vi "ATS_AsyncDMA_cFlags.vi"(7 "DeviceIn":i32, 8 "ReadSamples":T1, 10 "cFlags_Options":T2, 11 "Start Now / Wait":bool) -> (3 "cFlags_Out":u32 format="%.0x", 5 "DeviceOut":i32)   [LabVIEW 2010]
doc: "_____AlazarTech, Scope_____\n\nCreate the cFlags parameter on the StartAutoDMA and Asynchronous DMA transfer mode."
uses:
  ATS_ctl/ATS_AsyncDMA_cFlags_Opt.ctl
  ATS_ctl/ATS_ReadSamples.ctl
  ATS_ctl/ATS_Spec_Selector.ctl
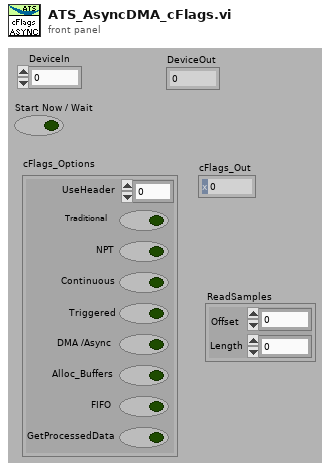
[diagram p1: front panel]
types:
  T1 = typedef "ATS_ReadSamples.ctl" = cluster{"Offset":i32, "Length":u32}
  T2 = typedef "ATS_AsyncDMA_cFlags_Opt.ctl" = cluster{"UseHeader":u32, "Traditional":bool, "NPT":bool, "Continuous":bool, "Triggered":bool, "DMA /Async":bool, "Alloc_Buffers":bool, "FIFO":bool, "GetProcessedData":bool}
  T3 = typedef "ATS_Spec_Selector.ctl" = enum16{"None", "ClckSource", "ClckEdge", "ClckRate", "InputRange", "InputCoupling", "Impedance", "Bandwidth", "AsyncDMA", "Memory", "ExtTrigCoupling", "ExtTrigRange", "AUX_IO_Trig", "AUX_IO_Slope", "Trigger_Source"}
  T4 = typedef "ATS_Global_Specs_Ctrl.ctl" = cluster{"ClckSource":cluster{"Internal":bool, "External":bool, "Medium Ext.":bool, "Slow Ext.":bool, "Ext. AC":bool, "Ext. DC":bool, "Ext. (PLL)":bool}, "ClckRate":cluster{"1 kS/s":bool, "2 kS/s":bool, "5 kS/s":bool, "10 kS/s":bool, "20 kS/s":bool, "50 kS/s":bool, "100 kS/s":bool, "200 kS/s":bool, "500 kS/s":bool, "1 MS/s":bool, "2 MS/s":bool, "5 MS/s":bool, "10 MS/s":bool, "20 MS/s":bool, "25 MS/s":bool, "50 MS/s":bool, "100 MS/s":bool, "125 MS/s":bool, "160 MS/s":bool, "180 MS/s":bool, "200 MS/s":bool, "250 MS/s":bool, "500 MS/s":bool, "1 GS/s":bool}, "ClckEdge":cluster{"Rising":bool, "Falling":bool}, "InputCoupling":cluster{"AC":bool, "DC":bool}, "InputRange":cluster{"20mV":bool, "40mV":bool, "50mV":bool, "80mV":bool, "100mV":bool, "200mV":bool, "400mV":bool, "500mV":bool, "800mV":bool, "1 V":bool, "2 V":bool, "4 V":bool, "5 V":bool, "8 V":bool, "10 V":bool, "16 V":bool, "20 V":bool, "40 V":bool, "HiFi":bool, "1.25 V":bool}, "Impedance":cluster{"1M ohms":bool, "50 ohms":bool, "300 ohms":bool}, "Bandwidth":cluster{"Full":bool, "Reduce":bool}, "RangeLim(50)":string, "AsyncDMA":cluster{"OnBoard":bool, "FPGA":bool}, "Memory":cluster{"VerifMem":bool, "HighMem":bool, "Combine":bool, "HighRecord":bool}, "ExtTrigCoupling":cluster{"AC":bool, "DC":bool}, "ExtTrigRange":cluster{"1 V":bool, "5 V":bool, "\nTTL":bool}, "AUX_IO_Trig":cluster{"Trig_Out":bool, "Trig_In":bool}, "AUX_IO_Slope":cluster{"Rising":bool, "Falling":bool}, "MaxPretrig":cluster{"MEM":u32, "FIFO":u32}, "AUX_I/O_Trig":cluster{"OUT_Trigger":bool, "OUT_PACER":bool, "OUT_BUSY":bool, "OUT_CLOCK":bool, "OUT_RESERVED":bool, "OUT_CAPTURE_ALMOST_DONE":bool, "OUT_AUXILIARY":bool, "OUT_SERIAL_DATA":bool, "IN_TRIGGER_ENABLE":bool, "IN_DIGITAL_TRIGGER":bool, "IN_GATE":bool, "IN_CAPTURE_ON_DEMAND":bool, "IN_RESET_TIMESTAMP":bool, "IN_SLOW_EXTERNAL_CLOCK":bool, "INPUT_AUXILIARY":bool, "INPUT_SERIAL_DATA":bool}, "ChannelsPerBoard":u8}
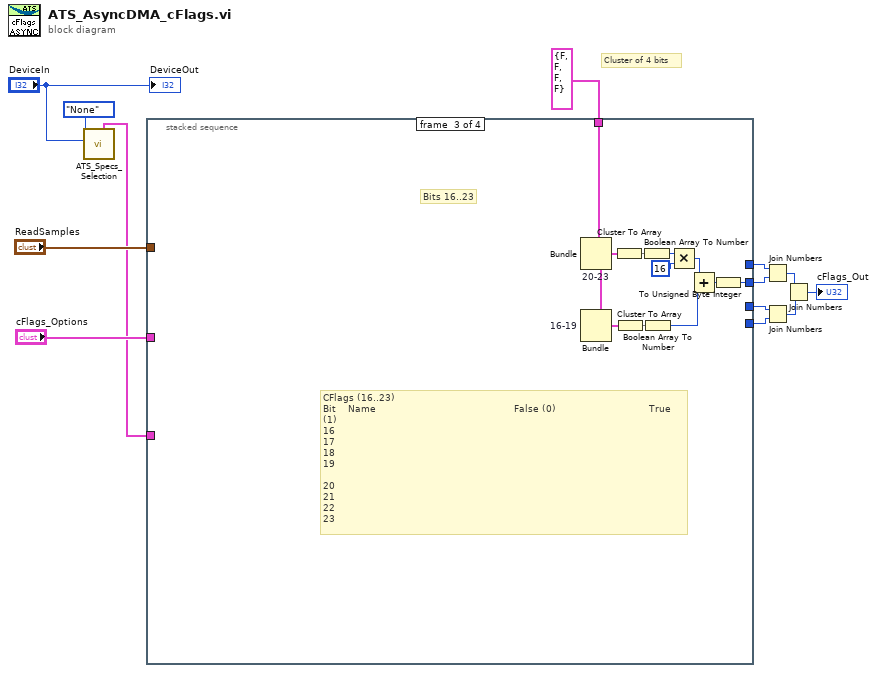
[diagram p0: block diagram]
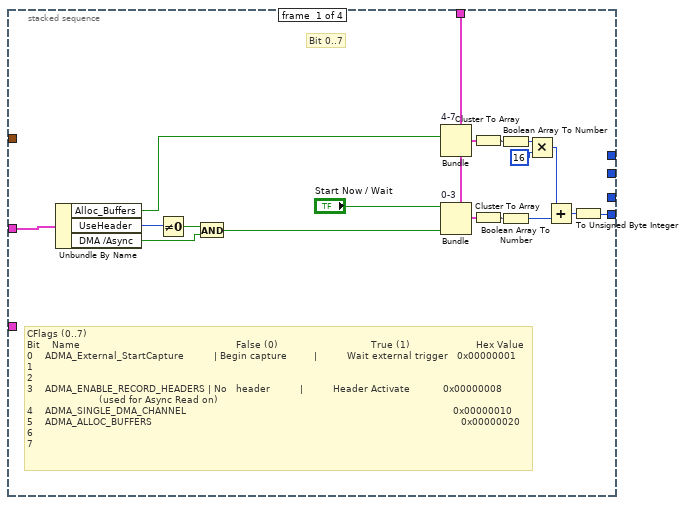
[diagram p2: hidden frame]
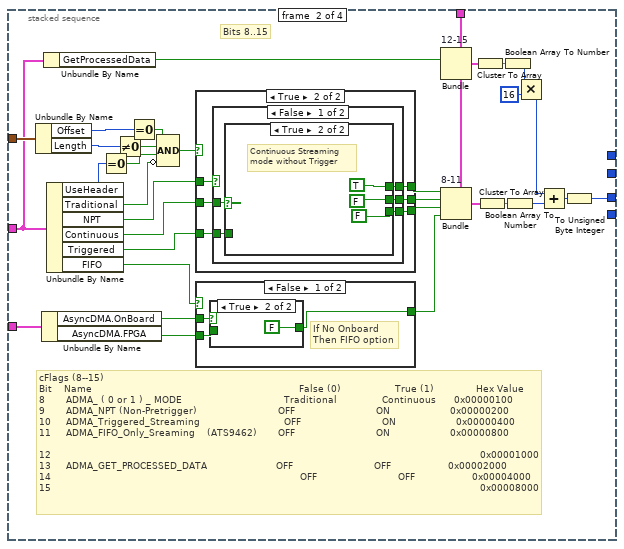
[diagram p3: hidden frame]
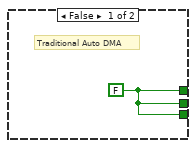
[diagram p6: hidden frame]
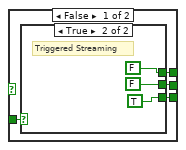
[diagram p7: hidden frame]
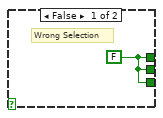
[diagram p8: hidden frame]
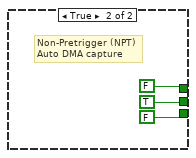
[diagram p9: hidden frame]
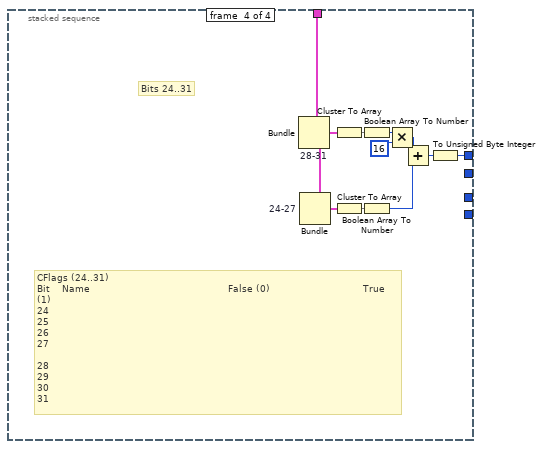
[diagram p10: hidden frame]
diagram:
  # "Cluster of 4 bits"
  n1 = call "ATS_Specs_Selection.vi"("Device"="DeviceIn", "ATS_Spec_Selector"=ATS_Spec_Selector."None") -> ("Specifications"=w2:T4)  [unwired: 3 in, 6 out]
  n2 = stacked-sequence {
    tunnel: cluster{bool, bool, bool, bool} {FALSE, FALSE, FALSE, FALSE} ("cluster") -> [w27 w53 w98 w109]
    tunnel: [w20 _ _ _] -> w11
    tunnel: [_ w61 _ _] -> w9
    tunnel: [_ _ _ w108] -> w7
    tunnel: [_ _ w97 _] -> w6
    tunnel: w2 -> [_ w42 _ _]
    tunnel: "cFlags_Options" -> [w19 w33 _ _]
    tunnel: "ReadSamples" -> [_ w50 _ _]
    frame #0 {
      # "CFlags (0..7)\nBit    Name                                                    False (0)                               True (1)                      Hex Value\n0    ADMA_External_StartCapture          | Begin capture         |          Wait external trigger   0x00000001\n1    \n2   \n3    ADMA_ENABLE_RECORD_HEADERS | No   header          |          Header Activate           0x00000008\n                        (used for Async Read on)\n4    ADMA_SINGLE_DMA_CHANNEL\t                                                                                       \t0x00000010\n5    ADMA_ALLOC_BUFFERS\t\t\t                                                                                                    0x00000020\n6\n7"
      # "Bit 0..7"
      n3 = Unbundle By Name(w19) -> ("Alloc_Buffers"=w14:bool, "UseHeader"=w18:u32, "DMA /Async"=w15:bool)
      n4 = Not Equal To 0?(x=w18) -> (x != 0?=w17:bool)
      n5 = And(x=w17, y=w15) -> (x .and. y?=w16:bool)
      n6 = Bundle "4-7"(cluster=w27, w14) -> (w28:cluster{bool, bool, bool, bool})  [unwired: 3 in]
      n7 = Bundle "0-3"(cluster=w27, "Start Now / Wait", w16) -> (w31:cluster{bool, bool, bool, bool})  [unwired: 2 in]
      n8 = Cluster To Array(cluster=w28) -> (array=w29:bool[])
      n9 = Cluster To Array(cluster=w31) -> (array=w30:bool[])
      n10 = Boolean Array To Number(Boolean array=w29) -> (number=w26:u32)
      n11 = Boolean Array To Number(Boolean array=w30) -> (number=w23:u32)
      n12 = Multiply(x=w26, y=u32 16) -> (x*y=w24:u32)
      n13 = Add(x=w24, y=w23) -> (x+y=w22:u32)
      n14 = To Unsigned Byte Integer(number=w22) -> (unsigned 8bit integer=w20:u8)
    }
    frame #1 {
      # "cFlags (8--15)\nBit    Name                                                                     False (0)                  True (1)              Hex Value\n8       ADMA_ ( 0 or 1 ) _ MODE                                  Traditional               Continuous      0x00000100\n9       ADMA_NPT (Non-Pretrigger)                           OFF                           ON                    0x00000200\n10     ADMA_Triggered_Streaming                            OFF                           ON                    0x00000400\n11     ADMA_FIFO_Only_Sreaming    (ATS9462)       OFF                           ON                    0x00000800\n\n12                                                                                                                                               0x00001000\n13     ADMA_GET_PROCESSED_DATA                       OFF                           OFF                   0x00002000\n14                                                                                   OFF                           OFF                   0x00004000\n15                                                                                                                                               0x00008000"
      # "Bits 8..15"
      n15 = Unbundle By Name(w50) -> ("Offset"=w49:i32, "Length"=w48:u32)
      n16 = Unbundle By Name(w42) -> ("AsyncDMA.OnBoard"=w38:bool, "AsyncDMA.FPGA"=w39:bool)
      n17 = Unbundle By Name(w33) -> ("GetProcessedData"=w32:bool)
      n18 = Unbundle By Name(w33) -> ("UseHeader"=w47:u32, "Traditional"=w46:bool, "NPT"=w43:bool, "Continuous"=w58:bool, "Triggered"=w45:bool, "FIFO"=w40:bool)
      n19 = Equal To 0?(x=w47) -> (x = 0?=w57:bool)
      n20 = Not Equal To 0?(x=w48) -> (x != 0?=w56:bool)
      n21 = Equal To 0?(x=w49) -> (x = 0?=w59:bool)
      n22 = Compound Arithmetic op=AND(w59, w56, w57, invert w46) -> (w60:bool)
      n23 = case shown="True" w60 {
        tunnel: w58 -> [_ w77]
        tunnel: [w71 w76] -> w52
        tunnel: [w71 w75] -> w51
        tunnel: [w71 w73] -> w44
        tunnel: w45 -> [_ w72]
        tunnel: w43 -> [_ w74]
        frame False {
          w71 = FALSE ("element")
          # "Traditional Auto DMA"
        }
        frame True {
          n24 = case shown="False" w74 {
            tunnel: w77 -> [w82 _]
            tunnel: [w81 FALSE ("element")] -> w76
            tunnel: [w80 TRUE ("element")] -> w75
            tunnel: [w79 FALSE ("Triggered")] -> w73
            tunnel: w72 -> [w78 _]
            frame False {
              n25 = case shown="True" w82 {
                tunnel: [w86 TRUE ("element")] -> w81
                tunnel: [w85 FALSE ("element")] -> w80
                tunnel: [w84 FALSE] -> w79
                tunnel: w78 -> [w83 _]
                frame False {
                  n26 = case shown="True" w83 {
                    tunnel: [w87 FALSE ("element")] -> w86
                    tunnel: [w87 FALSE ("element")] -> w85
                    tunnel: [w87 TRUE ("Triggered")] -> w84
                    frame False {
                      w87 = FALSE ("element")
                      # "Wrong Selection"
                    }
                    frame True {
                      # "Triggered Streaming"
                    }
                  }
                }
                frame True {
                  # "Continuous Streaming\nmode without Trigger"
                }
              }
            }
            frame True {
              # "Non-Pretrigger (NPT) \nAuto DMA capture"
            }
          }
        }
      }
      n27 = case shown="False" w40 {
        tunnel: [w66 w70] -> w41
        tunnel: w39 -> [w65 w70]
        tunnel: w38 -> [w67 _]
        frame False {
          # "If No Onboard\nThen FIFO option"
          n28 = case shown="True" w67 {
            tunnel: [w68 FALSE] -> w66
            tunnel: w65 -> [w68 _]
            frame False {
            }
            frame True {
            }
          }
        }
        frame True {
          # "FIFO available"
        }
      }
      n29 = Bundle "12-15"(cluster=w53, w32) -> (w63:cluster{bool, bool, bool, bool})  [unwired: 3 in]
      n30 = Bundle "8-11"(cluster=w53, w52, w51, w44, w41) -> (w54:cluster{bool, bool, bool, bool})
      n31 = Cluster To Array(cluster=w63) -> (array=w62:bool[])
      n32 = Cluster To Array(cluster=w54) -> (array=w55:bool[])
      n33 = Boolean Array To Number(Boolean array=w62) -> (number=w34:u32)
      n34 = Boolean Array To Number(Boolean array=w55) -> (number=w37:u32)
      n35 = Multiply(x=w34, y=u32 16) -> (x*y=w36:u32)
      n36 = Add(x=w36, y=w37) -> (x+y=w64:u32)
      n37 = To Unsigned Byte Integer(number=w64) -> (unsigned 8bit integer=w61:u8)
    }
    frame #2 {
      # "CFlags (16..23)\nBit    Name                                              False (0)                               True (1)\n16     \n17\n18\n19\n\n20\n21\n22\n23"
      # "Bits 16..23"
      n38 = Bundle "20-23"(cluster=w98) -> (w102:cluster{bool, bool, bool, bool})  [unwired: 4 in]
      n39 = Bundle "16-19"(cluster=w98) -> (w99:cluster{bool, bool, bool, bool})  [unwired: 4 in]
      n40 = Cluster To Array(cluster=w102) -> (array=w101:bool[])
      n41 = Cluster To Array(cluster=w99) -> (array=w100:bool[])
      n42 = Boolean Array To Number(Boolean array=w101) -> (number=w107:u32)
      n43 = Boolean Array To Number(Boolean array=w100) -> (number=w106:u32)
      n44 = Multiply(x=w107, y=u32 16) -> (x*y=w103:u32)
      n45 = Add(x=w103, y=w106) -> (x+y=w105:u32)
      n46 = To Unsigned Byte Integer(number=w105) -> (unsigned 8bit integer=w97:u8)
    }
    frame #3 {
      # "CFlags (24..31)\nBit    Name                                              False (0)                               True (1)\n24\n25\n26\n27\n\n28\n29\n30\n31"
      # "Bits 24..31"
      n47 = Bundle "28-31"(cluster=w109) -> (w110:cluster{bool, bool, bool, bool})  [unwired: 4 in]
      n48 = Bundle "24-27"(cluster=w109) -> (w113:cluster{bool, bool, bool, bool})  [unwired: 4 in]
      n49 = Cluster To Array(cluster=w110) -> (array=w111:bool[])
      n50 = Cluster To Array(cluster=w113) -> (array=w112:bool[])
      n51 = Boolean Array To Number(Boolean array=w111) -> (number=w116:u32)
      n52 = Boolean Array To Number(Boolean array=w112) -> (number=w117:u32)
      n53 = Multiply(x=w116, y=u32 16) -> (x*y=w115:u32)
      n54 = Add(x=w115, y=w117) -> (x+y=w118:u32)
      n55 = To Unsigned Byte Integer(number=w118) -> (unsigned 8bit integer=w108:u8)
    }
  }
  n56 = Join Numbers(hi=w7, lo=w6) -> ((hi.lo)=w12:u16)
  n57 = Join Numbers(hi=w9, lo=w11) -> ((hi.lo)=w10:u16)
  n58 = Join Numbers(hi=w12, lo=w10) -> ((hi.lo)=→"cFlags_Out":u32)
  "DeviceOut" <- "DeviceIn"
